vi "ActionVIOnCompile.vi"(8 "error in":errorcluster, 11 "Device Item Ref in":T14=18446744073709551615) -> (0 "error out":errorcluster)   [LabVIEW 2015, in "Fuel Injector Analysis Addon System Explorer.lvlib"]
uses:
  Fuel Injector Analysis Addon System Explorer.lvlib
  <vilib>/NI Veristand/Custom Device API/Custom Device Item Ref.ctl
  Shared/Types/Compiled.Settings.ctl
  Shared/Types/Injector info.ctl
  <vilib>/NI Veristand/Custom Device API/Waveform Data Reference.ctl
  <vilib>/NI Veristand/Custom Device API/Block Data Reference.ctl
  <vilib>/NI Veristand/Custom Device API/Data Reference.ctl
  Shared/Types/VS.Register.Info.ctl
  Shared/Types/Register.Info.ctl
  Shared/Types/FPGA Data Types.ctl
  Shared/Types/Shot.Parameters.ctl
  Shared/Types/Stage.Parameters.ctl
  Shared/Types/Stage.PullIn.Types.ctl
  Shared/Types/Stage.Transition.Types.ctl
  Shared/Types/Analysis.Channels.Select.ctl
  <vilib>/NI Veristand/Custom Device API/Data Access Type.ctl
  <vilib>/NI Veristand/Custom Device API/Custom Device Target Type.ctl
  Shared/Constants.vi
  <vilib>/NI Veristand/Custom Device Tools/Custom Device Utility Library/NI VeriStand - Search for Item by GUID.vi
  <vilib>/NI Veristand/Custom Device Tools/Custom Device Utility Library/NI VeriStand - Search for All Items by GUID.vi
  <vilib>/NI Veristand/Custom Device Tools/Custom Device Utility Library/NI VeriStand - Search for Item by Name.vi
  <vilib>/NI Veristand/Custom Device API/Get Item Property (Double).vi
  <vilib>/NI Veristand/Custom Device API/Get Item Property (U32).vi
  <vilib>/NI Veristand/Custom Device API/Set Item Property (Variant).vi
  Shared/Fuel Injector Analysis Addon Shared.lvlib
  <vilib>/NI Veristand/Custom Device API/Custom Device API.lvlib
  <vilib>/NI Veristand/Custom Device Tools/Custom Device Utility Library/Custom Device Utility Library.lvlib
  <vilib>/NI/NIVS Inline Async API/_Data Access System Explorer/Data Access System Explorer.lvlib
panel:
  out "output cluster":T1={"Name"="", "RIO.Address"="", "Bitfile.Path"=path "", "Injectors.Count"=0, "Rate.Hz"=0, "Injectors.Settings"=[], "Waveform.Refs"=[], "VS.Registers"={"Block Data refs"=[], "Values"=[]}, "Registers"=[], "Timing.Register"={"Name"="", "Data Type"=enum."<Null>", "Default Value"=variant(dbl 0.0)}, "Mux.Register"={"Name"="", "Data Type"=enum."<Null>", "Default Value"=variant(dbl 0.0)}, "Groups.Settings"=[]} {"Mux.Register"."Data Type" format="%.0x"; "Timing.Register"."Data Type" format="%.0x"; "Registers"."Register"."Data Type" format="%.0x"; "VS.Registers"."Block Data refs"."Data Reference" format="%.0x"}
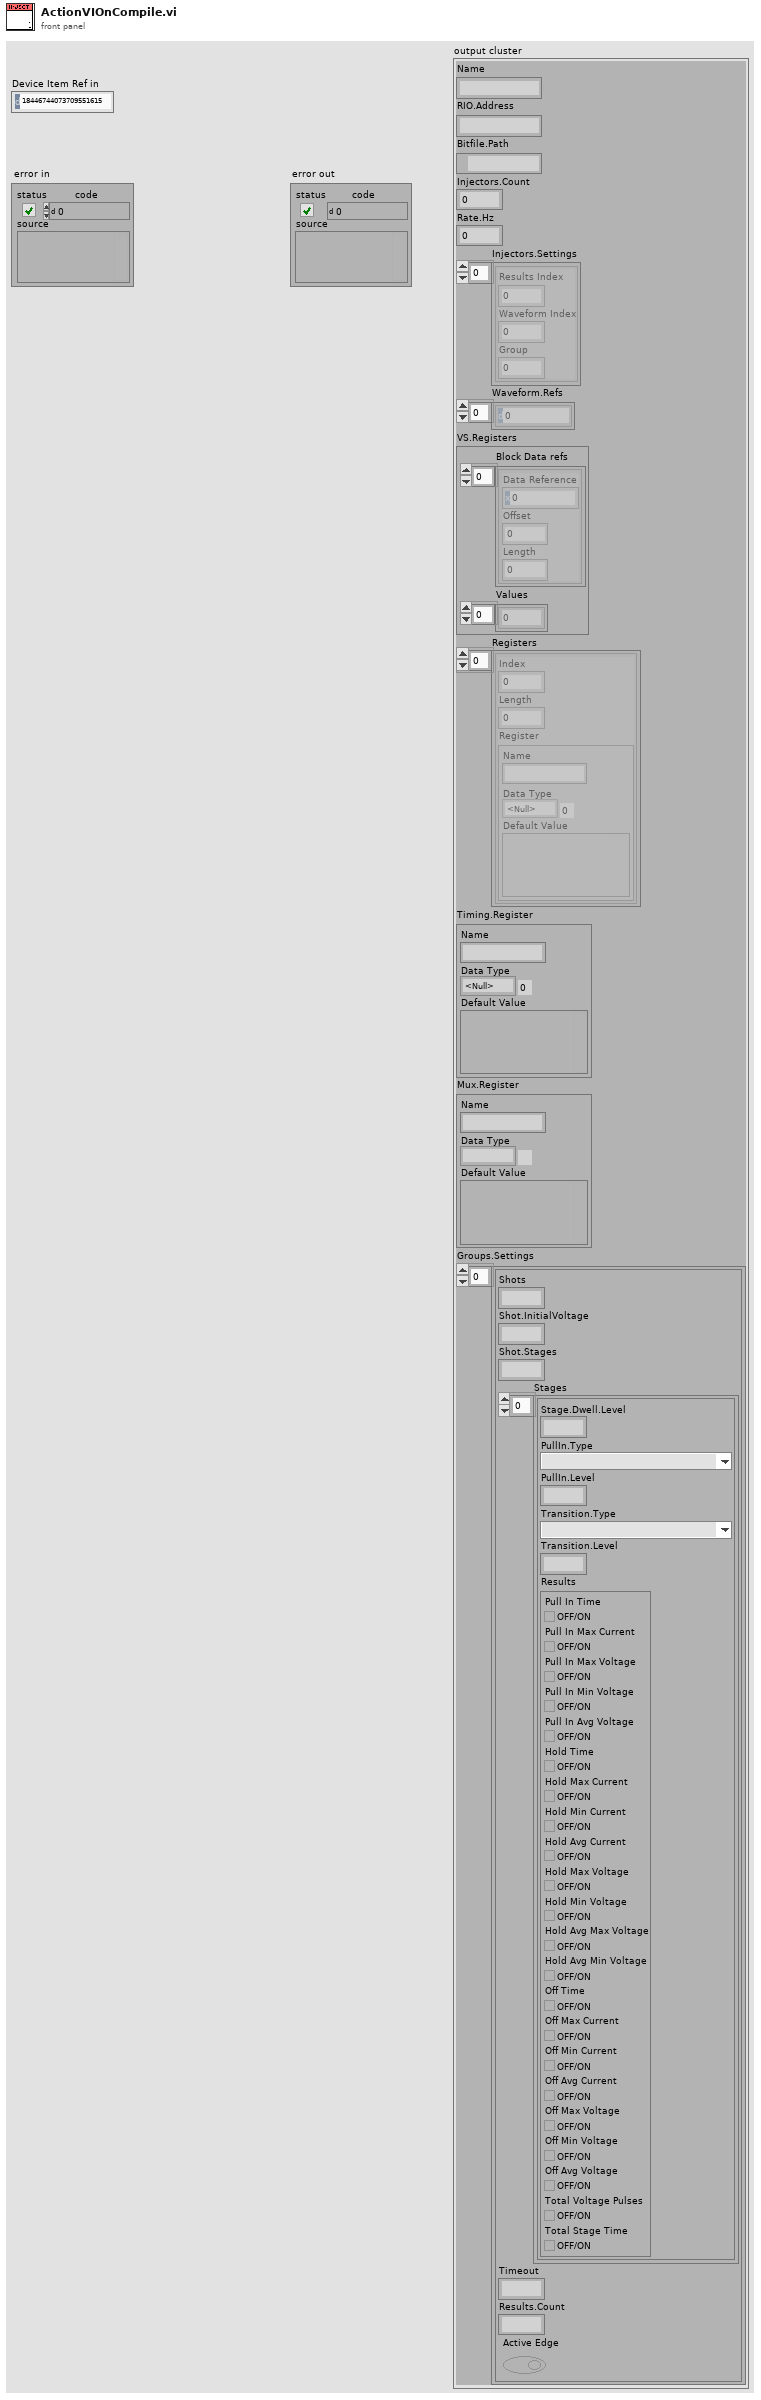
[diagram p1: front panel]
types:
  T1 = typedef "Fuel Injector Analysis Addon Shared.lvlib/Compiled.Settings.ctl" = cluster{"Name":string, "RIO.Address":string, "Bitfile.Path":path, "Injectors.Count":u32, "Rate.Hz":u32, "Injectors.Settings":T2[], "Waveform.Refs":T3[], "VS.Registers":cluster{"Block Data refs":T4[], "Values":dbl[]}, "Registers":T6[], "Timing.Register":T7, "Mux.Register":T7, "Groups.Settings":T9[]}
  T2 = typedef "Fuel Injector Analysis Addon Shared.lvlib/Injector info.ctl" = cluster{"Results Index":i32, "Waveform Index":i32, "Group":u16}
  T3 = typedef "Custom Device API.lvlib/Waveform Data Reference.ctl" = i32
  T4 = typedef "Custom Device API.lvlib/Block Data Reference.ctl" = cluster{"Data Reference":T5, "Offset":u64, "Length":u64}
  T5 = typedef "Custom Device API.lvlib/Data Reference.ctl" = i32
  T6 = typedef "Fuel Injector Analysis Addon Shared.lvlib/VS.Register.Info.ctl" = cluster{"Index":i32, "Length":i32, "Register":T7}
  T7 = typedef "Fuel Injector Analysis Addon Shared.lvlib/Register.Info.ctl" = cluster{"Name":string, "Data Type":T8, "Default Value":variant}
  T8 = typedef "Fuel Injector Analysis Addon Shared.lvlib/FPGA Data Types.ctl" = enum8{"<Null>", "Injector.Core.Setting", "Injector.Global.Setting", "Injector.Mux.Setting", "Injector.Timing"}
  T9 = typedef "Fuel Injector Analysis Addon Shared.lvlib/Shot.Parameters.ctl" = cluster{"Shots":u32, "Shot.InitialVoltage":dbl, "Shot.Stages":u32, "Stages":T10[], "Timeout":dbl, "Results.Count":i32, "Active Edge":bool}
  T10 = typedef "Fuel Injector Analysis Addon Shared.lvlib/Stage.Parameters.ctl" = cluster{"Stage.Dwell.Level":dbl, "PullIn.Type":T11, "PullIn.Level":dbl, "Transition.Type":T12, "Transition.Level":dbl, "Results":T13}
  T11 = typedef "Fuel Injector Analysis Addon Shared.lvlib/Stage.PullIn.Types.ctl" = enum8{"Pull In Transition Pulses", "Pull In Transition Current Drop"}
  T12 = typedef "Fuel Injector Analysis Addon Shared.lvlib/Stage.Transition.Types.ctl" = enum8{"Stage Transition Inactive Time", "Stage Transition Voltage Increase", "Stage Transition Current Decrease", "Stage Transition Active Time"}
  T13 = typedef "Fuel Injector Analysis Addon Shared.lvlib/Analysis.Channels.Select.ctl" = cluster{"Pull In Time":bool, "Pull In Max Current":bool, "Pull In Max Voltage":bool, "Pull In Min Voltage":bool, "Pull In Avg Voltage":bool, "Hold Time":bool, "Hold Max Current":bool, "Hold Min Current":bool, "Hold Avg Current":bool, "Hold Max Voltage":bool, "Hold Min Voltage":bool, "Hold Avg Max Voltage":bool, "Hold Avg Min Voltage":bool, "Off Time":bool, "Off Max Current":bool, "Off Min Current":bool, "Off Avg Current":bool, "Off Max Voltage":bool, "Off Min Voltage":bool, "Off Avg Voltage":bool, "Total Voltage Pulses":bool, "Total Stage Time":bool}
  T14 = typedef "Custom Device API.lvlib/Custom Device Item Ref.ctl" = u64
  T15 = enum16{"Output/Write", "Input/Read", "Input/ReadWrite"}
  T16 = typedef "Custom Device API.lvlib/Custom Device Target Type.ctl" = enum16{"PharLap", "VxWorks", "Windows", "Linux_32_ARM", "Linux_x64"}
  T17 = typedef "Custom Device API.lvlib/Data Access Type.ctl" = enum16{"Read", "Write"}
  T18 = cluster{"Name":string, "Type":enum16{"Output/Write", "Input/Read", "Input/ReadWrite"}, "VS Refs":T14[]}
  T19 = typedef "Custom Device API.lvlib/Custom Device Item Info.ctl" = cluster{"Name":string, "Is Channel":bool, "GUID":string, "Is Waveform":bool}
  T20 = typedef "Fuel Injector Analysis Addon Shared.lvlib/Main Settings.ctl" = cluster{"RIO Device Address":string, "Local bitfile path":path, "RT bitfile path":path, "Number of injectors":u16, "Sample rate (S/s)":u32}
  T21 = typedef "Custom Device API.lvlib/Custom Device Channel.ctl" = cluster{"Type":T22, "Units":string, "Default Value":dbl, "Faultable":bool, "Scalable":bool}
  T22 = typedef "Custom Device API.lvlib/Custom Device Channel Type.ctl" = enum16{"Input", "Output"}
  T23 = cluster{"Name":string, "Type":enum16{"Output/Write", "Input/Read", "Input/ReadWrite"}, "VS Refs":T14[]}[]
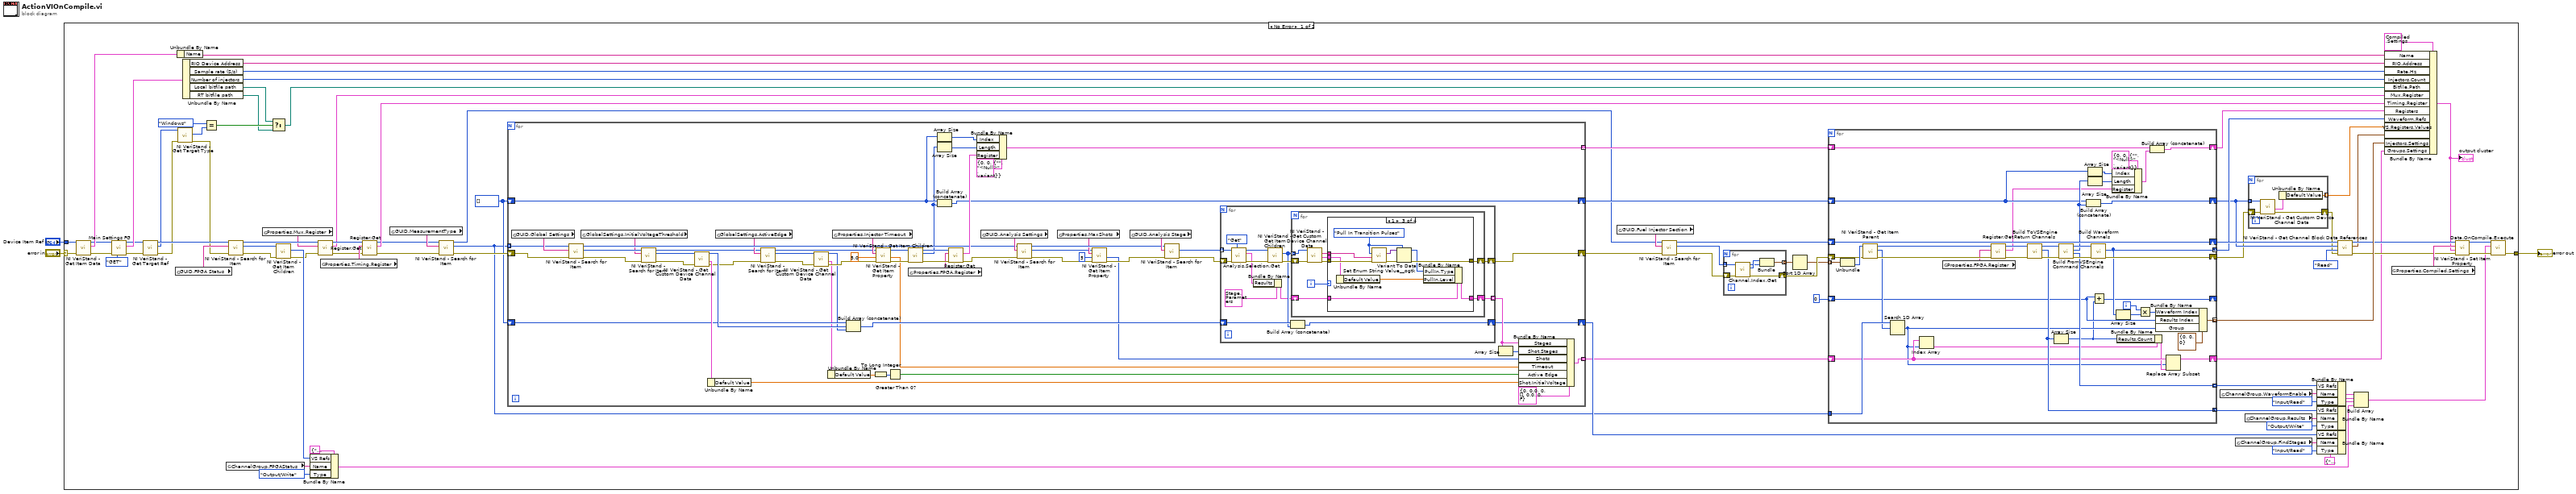
[diagram p0: block diagram]
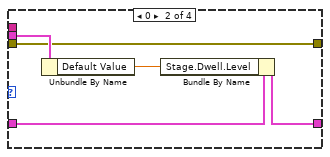
[diagram p3: hidden frame]
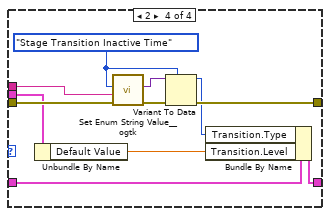
[diagram p4: hidden frame]
diagram:
  n1 = case shown="No Error" "error in" {
    selector: "error in" -> [w92 w260]
    tunnel: "Device Item Ref in" -> [w91 _]
    tunnel: [w79 w260] -> w1
    frame No Error {
      w9 = T14[] []
      w22 = T18 {"Name"="", "Type"=enum."Input/Read", "VS Refs"=[]} ("Group")
      n2 = call <vilib>:"NI VeriStand - Get Item Data.vi"("error in (no error)"=w92, "Item Ref in"=w91) -> ("error out"=w88:errorcluster, "Item Info"=w90:T19, "Item Ref out"=w87:T14)  [unwired: 6 in, 1 out]
      n3 = call "Main Settings FG.vi"("Action"=enum8{"GET", "SET"}."GET", "error in (no error)"=w88, "Item Ref"=w87) -> ("error out"=w42:errorcluster, "Main Settings out"=w86:T20, "Item Ref out"=w61:T14)  [unwired: 6 in]
      n4 = call <vilib>:"NI VeriStand - Get Target Ref.vi"("error in"=w42, "Item Ref in"=w61) -> ("error out"=w40:errorcluster, "Target Ref"=w41:T14, "Item Ref out"=w43:T14)  [unwired: 6 in, 1 out]
      n5 = global read "Constants.vi" "GUID.FPGA Status"() -> (w60:string)
      n6 = Unbundle By Name(w90) -> ("Name"=w89:string)
      n7 = call <vilib>:"NI VeriStand - Get Target Type.vi"("error in (no error)"=w40, "Item Ref in"=w41) -> ("error out"=w39:errorcluster, "Target Type"=w38:T16)  [unwired: 7 in, 1 out]
      n8 = Unbundle By Name(w86) -> ("RIO Device Address"=w85:string, "Sample rate (S/s)"=w82:u32, "Number of injectors"=w74:u16, "Local bitfile path"=w34:path, "RT bitfile path"=w35:path)
      n9 = Equal?(x=Custom_Device_Target_Type."Windows", y=w38) -> (x = y?=w36:bool)
      n10 = global read "Constants.vi" "ChannelGroup.FPGAStatus"() -> (w57:string)
      n11 = call-poly <vilib>:"NI VeriStand - Search for Item.vi"("error in"=w39, "Item GUID"=w60, "Section Ref in"=w43) -> ("error out"=w55:errorcluster, "Item Ref"=w59:T14, "Section Ref out"=w52:T14)  [unwired: 5 in, 1 out]
      n12 = global read "Constants.vi" "Properties.Mux.Register"() -> (w48:string)
      n13 = Select(t=w34, s=w36, f=w35) -> (s? t:f=w33:path)
      n14 = call <vilib>:"NI VeriStand - Get Item Children.vi"("error in (no error)"=w55, "Item Ref in"=w59) -> ("error out"=w50:errorcluster, "Child Refs"=w56:T14[])  [unwired: 6 in, 2 out]
      n15 = Bundle By Name(cluster=T18 {"Name"="", "Type"=enum."Input/Read", "VS Refs"=[]} ("Group"), "VS Refs"=w56, "Name"=w57, "Type"=T15."Output/Write") -> (w54:T18)
      n16 = call "Register.Get.vi"("error in (no error)"=w50, "Property"=w48, "Section Ref in"=w52) -> ("error out"=w49:errorcluster, "Register"=w47:T7, "Item Ref out"=w51:T14)  [unwired: 6 in]
      n17 = global read "Constants.vi" "Properties.Timing.Register"() -> (w53:string)
      n18 = call "Register.Get.vi"("error in (no error)"=w49, "Property"=w53, "Section Ref in"=w51) -> ("error out"=w14:errorcluster, "Register"=w62:T7, "Item Ref out"=w11:T14)  [unwired: 6 in]
      n19 = global read "Constants.vi" "GUID.MeasurementType"() -> (w12:string)
      n20 = call-poly <vilib>:"NI VeriStand - Search for Item.vi"("error in"=w14, "Item GUID"=w12, "Section Ref in"=w11) -> ("error out"=w13:errorcluster, "Item Refs"=w8:T14[], "Section Ref out"=w7:T14)  [unwired: 5 in, 1 out]
      n21 = for {
        tunnel: [w112] -> w66 mode=indexing
        shift-right: [w147] -> w26
        shift-left: w13 -> [w119]
        shift-right: [w120] -> w21
        shift-left: w9 -> [w116]
        shift-right: [w110] -> w67
        shift-left: w9 -> [w114]
        tunnel: w8 -> [w109] mode=indexing
        tunnel: [w108] -> w6 mode=indexing
        n22 = global read "Constants.vi" "GUID.Global Settings"() -> (w154:string)
        n23 = call-poly <vilib>:"NI VeriStand - Search for Item.vi"("error in"=w119, "Item GUID"=w154, "Section Ref in"=w109) -> ("error out"=w128:errorcluster, "Item Ref"=w127:T14, "Section Ref out"=w136:T14)  [unwired: 5 in, 1 out]
        n24 = global read "Constants.vi" "GlobalSettings.InitialVoltageThreshold"() -> (w126:string)
        n25 = call-poly <vilib>:"NI VeriStand - Search for Item.vi"("error in"=w128, "Item Name"=w126, "Section Ref in"=w127) -> ("error out"=w123:errorcluster, "Item Ref"=w122:T14, "Section Ref out"=w103:T14)  [unwired: 5 in, 1 out]
        n26 = call <vilib>:"NI VeriStand - Get Custom Device Channel Data.vi"("error in (no error)"=w123, "Channel Ref in"=w122) -> ("error out"=w102:errorcluster, "Channel"=w124:T21, "Channel Ref out"=w121:T14)  [unwired: 4 in, 3 out]
        n27 = Unbundle By Name(w124) -> ("Default Value"=w117:dbl)
        n28 = global read "Constants.vi" "GlobalSettings.ActiveEdge"() -> (w104:string)
        n29 = call-poly <vilib>:"NI VeriStand - Search for Item.vi"("error in"=w102, "Item Name"=w104, "Section Ref in"=w103) -> ("error out"=w105:errorcluster, "Item Ref"=w106:T14, "Section Ref out"=w95:T14)  [unwired: 5 in, 1 out]
        n30 = call <vilib>:"NI VeriStand - Get Custom Device Channel Data.vi"("error in (no error)"=w105, "Channel Ref in"=w106) -> ("error out"=w101:errorcluster, "Channel"=w99:T21, "Channel Ref out"=w100:T14)  [unwired: 4 in, 3 out]
        n31 = Unbundle By Name(w99) -> ("Default Value"=w98:dbl)
        n32 = global read "Constants.vi" "Properties.Injector Timeout"() -> (w143:string)
        n33 = Build Array (concatenate)(w116, w121, w100) -> (w125:T14[])
        n34 = To Long Integer(number=w98) -> (32bit integer=w97:i32)
        n35 = call-poly <vilib>:"NI VeriStand - Get Item Property.vi"("error in (no error)"=w101, "Default Value"=5.0, "Property Name"=w143, "Item Ref in"=w95) -> ("error out"=w142:errorcluster, "Value"=w107:dbl, "Item Ref out"=w141:T14)  [unwired: 4 in, 1 out]
        n36 = Greater Than 0?(x=w97) -> (x > 0?=w96:bool)
        n37 = call <vilib>:"NI VeriStand - Get Item Children.vi"("error in (no error)"=w142, "Item Ref in"=w141) -> ("error out"=w152:errorcluster, "Child Refs"=w111:T14[], "Item Ref out"=w149:T14)  [unwired: 6 in, 1 out]
        n38 = global read "Constants.vi" "Properties.FPGA.Register"() -> (w148:string)
        n39 = Array Size(array=w114) -> (size(s)=w113:i32)
        n40 = Array Size(array=w111) -> (size(s)=w115:i32)
        n41 = Build Array (concatenate)(w114, w111) -> (w110:T14[])
        n42 = call "Register.Get.vi"("error in (no error)"=w152, "Property"=w148, "Section Ref in"=w149) -> ("error out"=w134:errorcluster, "Register"=w150:T7)  [unwired: 6 in, 1 out]
        n43 = Bundle By Name(cluster=T6 {"Index"=0, "Length"=0, "Register"={"Name"="", "Data Type"=enum."<Null>", "Default Value"=variant}} ("Cluster"), "Index"=w113, "Length"=w115, "Register"=w150) -> (w112:T6)
        n44 = global read "Constants.vi" "GUID.Analysis Settings"() -> (w137:string)
        n45 = call-poly <vilib>:"NI VeriStand - Search for Item.vi"("error in"=w134, "Item GUID"=w137, "Section Ref in"=w136) -> ("error out"=w130:errorcluster, "Item Ref"=w131:T14, "Section Ref out"=w135:T14)  [unwired: 5 in, 1 out]
        n46 = global read "Constants.vi" "Properties.MaxShots"() -> (w132:string)
        n47 = call-poly <vilib>:"NI VeriStand - Get Item Property.vi"("error in (no error)"=w130, "Default Value"=u32 5, "Property Name"=w132, "Item Ref in"=w131) -> ("error out"=w129:errorcluster, "Value"=w118:u32)  [unwired: 4 in, 2 out]
        n48 = global read "Constants.vi" "GUID.Analysis Stage"() -> (w153:string)
        n49 = call-poly <vilib>:"NI VeriStand - Search for Item.vi"("error in"=w129, "Item GUID"=w153, "Section Ref in"=w135) -> ("error out"=w146:errorcluster, "Item Refs"=w145:T14[])  [unwired: 5 in, 2 out]
        n50 = for {
          tunnel: w145 -> [w167] mode=indexing
          shift-right: [w162] -> w147
          shift-left: w146 -> [w168]
          tunnel: [w161] -> w139 mode=indexing
          shift-right: [w158] -> w120
          shift-left: w125 -> [w160]
          n51 = call "Analysis.Selection.Get.vi"("Action"=enum8{"Get", "Set"}."Get", "error in (no error)"=w168, "Item Ref in"=w167) -> ("error out"=w165:errorcluster, "Selections"=w155:T13, "Item Ref out"=w163:T14)  [unwired: 6 in]
          n52 = Bundle By Name(cluster=T10 {"Stage.Dwell.Level"=0.0, "PullIn.Type"=enum."Pull In Transition Pulses", "PullIn.Level"=0.0, "Transition.Type"=enum."Stage Transition Voltage Increase", "Transition.Level"=0.0, "Results"={"Pull In Time"=TRUE, "Pull In Max Current"=TRUE, "Pull In Max Voltage"=TRUE, "Pull In Min Voltage"=TRUE, "Pull In Avg Voltage"=TRUE, "Hold Time"=TRUE, "Hold Max Current"=TRUE, "Hold Min Current"=TRUE, "Hold Avg Current"=TRUE, "Hold Max Voltage"=TRUE, "Hold Min Voltage"=TRUE, "Hold Avg Max Voltage"=TRUE, "Hold Avg Min Voltage"=TRUE, "Off Time"=TRUE, "Off Max Current"=TRUE, "Off Min Current"=TRUE, "Off Avg Current"=TRUE, "Off Max Voltage"=TRUE, "Off Min Voltage"=TRUE, "Off Avg Voltage"=TRUE, "Total Voltage Pulses"=TRUE, "Total Stage Time"=TRUE}}, "Results"=w155) -> (w156:T10)
          n53 = call <vilib>:"NI VeriStand - Get Item Children.vi"("error in (no error)"=w165, "Item Ref in"=w163) -> ("error out"=w164:errorcluster, "Child Refs"=w159:T14[])  [unwired: 6 in, 2 out]
          n54 = Build Array (concatenate)(w160, w159) -> (w158:T14[])
          n55 = for {
            shift-right: [w171] -> w162
            shift-left: w164 -> [w177]
            tunnel: w159 -> [w176] mode=indexing
            shift-right: [w169] -> w161
            shift-left: w156 -> [w170]
            i -> [w174]
            n56 = call <vilib>:"NI VeriStand - Get Custom Device Channel Data.vi"("error in (no error)"=w177, "Channel Ref in"=w176) -> ("error out"=w175:errorcluster, "Channel"=w173:T21, "Channel Name"=w172:string)  [unwired: 4 in, 3 out]
            n57 = case shown="1" w174 {
              tunnel: w175 -> [w179 w183 w195 w206]
              tunnel: w173 -> [_ w184 w190 w200]
              tunnel: w172 -> [_ _ w194 w205]
              tunnel: [w179 w183 w189 w201] -> w171
              tunnel: w170 -> [w178 w182 w188 w198]
              tunnel: [w178 w180 w187 w197] -> w169
              frame Default {
              }
              frame 0 {
                n58 = Unbundle By Name(w184) -> ("Default Value"=w181:dbl)
                n59 = Bundle By Name(cluster=w182, "Stage.Dwell.Level"=w181) -> (w180:T10)
              }
              frame 1 {
                w191 = Stage.PullIn.Types."Pull In Transition Pulses" ("PullIn.Type")
                n60 = Unbundle By Name(w190) -> ("Default Value"=w185:dbl)
                n61 = call <userlib>:"Set Enum String Value__ogtk.vi"("error in (no error)"=w195, "String Value"=w194, "Default Enum Value"=w191) -> ("error out"=w193:errorcluster, "Enum"=w192:variant)  [unwired: 7 in]
                n62 = Variant To Data(error in=w193, type=w191, Variant=w192) -> (data=w186:T11, error out=w189:errorcluster)
                n63 = Bundle By Name(cluster=w188, "PullIn.Type"=w186, "PullIn.Level"=w185) -> (w187:T10)
              }
              frame 2 {
                w202 = Stage.Transition.Types."Stage Transition Inactive Time" ("Stage.Transition")
                n64 = Unbundle By Name(w200) -> ("Default Value"=w199:dbl)
                n65 = call <userlib>:"Set Enum String Value__ogtk.vi"("error in (no error)"=w206, "String Value"=w205, "Default Enum Value"=w202) -> ("error out"=w204:errorcluster, "Enum"=w203:variant)  [unwired: 7 in]
                n66 = Variant To Data(error in=w204, type=w202, Variant=w203) -> (data=w196:T12, error out=w201:errorcluster)
                n67 = Bundle By Name(cluster=w198, "Transition.Type"=w196, "Transition.Level"=w199) -> (w197:T10)
              }
            }
          }
        }
        n68 = Array Size(array=w139) -> (size(s)=w138:i32)
        n69 = Bundle By Name(cluster=T9 {"Shots"=0, "Shot.InitialVoltage"=0.0, "Shot.Stages"=0, "Stages"=[], "Timeout"=0.0, "Results.Count"=0, "Active Edge"=FALSE} ("Parameters"), "Stages"=w139, "Shot.Stages"=w138, "Shots"=w118, "Timeout"=w107, "Active Edge"=w96, "Shot.InitialVoltage"=w117) -> (w108:T9)
      }
      n70 = global read "Constants.vi" "GUID.Fuel Injector Section"() -> (w84:string)
      n71 = call-poly <vilib>:"NI VeriStand - Search for Item.vi"("error in"=w26, "Item GUID"=w84, "Section Ref in"=w7) -> ("error out"=w18:errorcluster, "Item Refs"=w19:T14[], "Section Ref out"=w83:T14)  [unwired: 5 in, 1 out]
      n72 = for {
        tunnel: w19 -> [w212] mode=indexing
        shift-right: [w210] -> w17
        shift-left: w18 -> [w211]
        tunnel: [w207] -> w16 mode=indexing
        n73 = call "Channel.Index.Get.vi"("error in (no error)"=w211, "Ref in"=w212) -> ("error out"=w210:errorcluster, "Value"=w209:u16, "Ref out"=w208:T14)  [unwired: 6 in, 1 out]
        n74 = Bundle("Value"=w209, "Ref out"=w208) -> (w207:cluster{"Value":u16, "Ref out":T14})  [unwired: 1 in]
      }
      n75 = Sort 1D Array(array=w16) -> (sorted array=w15:cluster{"Value":u16, "Ref out":T14}[])
      n76 = for {
        shift-right: [w252] -> w28
        shift-left: w17 -> [w226]
        tunnel: [w241] -> w75 mode=indexing
        tunnel: [w243] -> w44 mode=concatenating
        shift-right: [w251] -> w45
        shift-left: w83 -> [w251]
        tunnel: [w248] -> w73 mode=concatenating
        tunnel: [w244] -> w72 mode=indexing
        shift-right: [w234] -> w30
        shift-left: w67 -> [w235]
        shift-right: [w233] -> w63
        shift-left: w66 -> [w238]
        tunnel: w15 -> [w229] mode=indexing
        tunnel: w8 -> [w224]
        shift-right: [w218] -> w10
        shift-left: w6 -> [w220]
        shift-right: [w213] -> _
        shift-left: 0 -> [w215]
        i -> [w247]
        n77 = Unbundle(w229) -> ("Ref out"=w228:T14)  [unwired: 1 out]
        n78 = call <vilib>:"NI VeriStand - Get Item Parent.vi"("error in (no error)"=w226, "Item Ref in"=w228) -> ("error out"=w225:errorcluster, "Parent Ref"=w223:T14, "Item Ref out"=w227:T14)  [unwired: 6 in, 1 out]
        n79 = Search 1D Array(1D array=w224, element=w223) -> (index of element=w217:i32)  [unwired: 1 in]
        n80 = Index Array(array=w220, index=w217) -> (element=w222:T9)
        n81 = global read "Constants.vi" "Properties.FPGA.Register"() -> (w221:string)
        n82 = call "Register.Get.vi"("error in (no error)"=w225, "Property"=w221, "Section Ref in"=w227) -> ("error out"=w232:errorcluster, "Register"=w230:T7, "Item Ref out"=w231:T14)  [unwired: 6 in]
        n83 = call "Build ToVSEngine Return Channels.vi"("error in (no error)"=w232, "Injector section ref in"=w231) -> ("error out"=w254:errorcluster, "Results"=w248:T14[], "Injector section ref out"=w249:T14)  [unwired: 7 in]
        n84 = Array Size(array=w248) -> (size(s)=w214:i32)
        n85 = call "Build FromVSEngine Command Channels.vi"("error in (no error)"=w254, "Injector section ref in"=w249) -> ("error out"=w253:errorcluster, "WaveformEnable?"=w241:T14, "InjectionSettings"=w236:T14[], "Injector section ref out"=w242:T14)  [unwired: 6 in]
        n86 = Build Array (concatenate)(w235, w236) -> (w234:T14[])
        n87 = Array Size(array=w235) -> (size(s)=w239:i32)
        n88 = Array Size(array=w236) -> (size(s)=w216:i32)
        n89 = call "Build Waveform Channels.vi"("error in (no error)"=w253, "Injector section ref in"=w242) -> ("error out"=w252:errorcluster, "Waveform channel array out"=w243:T3[])  [unwired: 7 in, 1 out]
        n90 = Add(x=w215, y=w214) -> (x+y=w213:i32)
        n91 = Bundle By Name(cluster=T6 {"Index"=0, "Length"=0, "Register"={"Name"="", "Data Type"=enum."<Null>", "Default Value"=variant}} ("Cluster"), "Index"=w239, "Length"=w216, "Register"=w230) -> (w237:T6)
        n92 = Array Size(array=w243) -> (size(s)=w250:i32)
        n93 = Bundle By Name(cluster=w222, "Results.Count"=w214) -> (w219:T9)
        n94 = Multiply(x=w247, y=w250) -> (x*y=w245:i32)
        n95 = Build Array (concatenate)(w238, w237) -> (w233:T6[])
        n96 = Bundle By Name(cluster=T2 {"Results Index"=0, "Waveform Index"=0, "Group"=0} ("Injector info"), "Waveform Index"=w245, "Results Index"=w215, "Group"=w217) -> (w244:T2)
        n97 = Replace Array Subset(array=w220, new element=w219, index=w217) -> (w218:T9[])
      }
      n98 = global read "Constants.vi" "ChannelGroup.WaveformEnable"() -> (w76:string)
      n99 = global read "Constants.vi" "ChannelGroup.FindStages"() -> (w23:string)
      n100 = global read "Constants.vi" "ChannelGroup.Results"() -> (w77:string)
      n101 = for {
        tunnel: w30 -> [w259] mode=indexing
        shift-right: [w257] -> w27
        shift-left: w28 -> [w258]
        tunnel: [w255] -> w29 mode=indexing
        n102 = call <vilib>:"NI VeriStand - Get Custom Device Channel Data.vi"("error in (no error)"=w258, "Channel Ref in"=w259) -> ("error out"=w257:errorcluster, "Channel"=w256:T21)  [unwired: 4 in, 4 out]
        n103 = Unbundle By Name(w256) -> ("Default Value"=w255:dbl)
      }
      n104 = Bundle By Name(cluster=w22, "VS Refs"=w75, "Name"=w76, "Type"=T15."Input/Read") -> (w70:T18)
      n105 = Bundle By Name(cluster=w22, "VS Refs"=w73, "Name"=w77, "Type"=T15."Output/Write") -> (w71:T18)
      n106 = Bundle By Name(cluster=w22, "VS Refs"=w21, "Name"=w23, "Type"=T15."Input/Read") -> (w20:T18)
      n107 = call <vilib>:"NI VeriStand - Get Channel Block Data References.vi"("error in (no error)"=w27, "Access"=Data_Access_Type."Read", "Channel Refs"=w30, "Device Ref in"=w45) -> ("error out"=w64:errorcluster, "Block Data Refs"=w5:T4[], "Device Ref out"=w46:T14)  [unwired: 4 in, 1 out]
      n108 = Build Array(w70, w71, w20, w54) -> (w31:T23)
      n109 = Bundle By Name(cluster=T1 {"Name"="", "RIO.Address"="", "Bitfile.Path"=path "", "Injectors.Count"=0, "Rate.Hz"=0, "Injectors.Settings"=[], "Waveform.Refs"=[], "VS.Registers"={"Block Data refs"=[], "Values"=[]}, "Registers"=[], "Timing.Register"={"Name"="", "Data Type"=enum."<Null>", "Default Value"=variant(dbl 0.0)}, "Mux.Register"={"Name"="", "Data Type"=enum."<Null>", "Default Value"=variant(dbl 0.0)}, "Groups.Settings"=[]} ("Settings.Compiled"), "Name"=w89, "RIO.Address"=w85, "Rate.Hz"=w82, "Injectors.Count"=w74, "Bitfile.Path"=w33, "Mux.Register"=w47, "Timing.Register"=w62, "Registers"=w63, "Waveform.Refs"=w44, "VS.Registers.Values"=w29, "VS.Registers.Block Data refs"=w5, "Injectors.Settings"=w72, "Groups.Settings"=w10) -> (w32:T1)
      "output cluster" <- w32
      n110 = global read "Constants.vi" "Properties.Compiled.Settings"() -> (w94:string)
      n111 = call-poly <vilib>:"NI VeriStand - Set Item Property.vi"("error in (no error)"=w64, "Value"=w32, "Property Name"=w94, "Item Ref in"=w46) -> ("error out"=w80:errorcluster, "Item Ref out"=w78:T14)  [unwired: 5 in, 1 out]
      n112 = call <vilib>:"Data.OnCompile.Execute.vi"("error in"=w80, "VS Ref Groups"=w31, "Custom Device Ref"=w78) -> ("error out"=w79:errorcluster)  [unwired: 7 in, 1 out]
    }
    frame Error {
    }
  }
  "error out" <- w1
